vi "Write Single Holding Register.vi"(8 "error in (no error)":errorcluster, 9 "register to write":u16, 10 "address":u16, 11 "Modbus instance in":refnum<class "Modbus API.lvclass">) -> (0 "error out":errorcluster, 3 "Modbus instance out":refnum<class "Modbus API.lvclass">)   [LabVIEW 2020, in "SubVIs.lvlib" / "Modbus API.lvclass"]
doc: "Writes <B>register to write</B> to <B>address</B> of the device."
uses:
  <vilib>/Modbus/subvis/Modbus API/Modbus API.lvclass
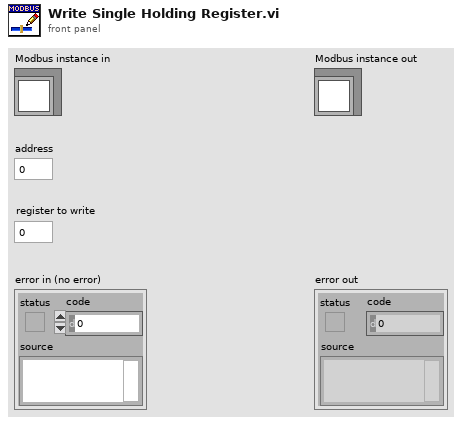
[diagram p1: front panel]
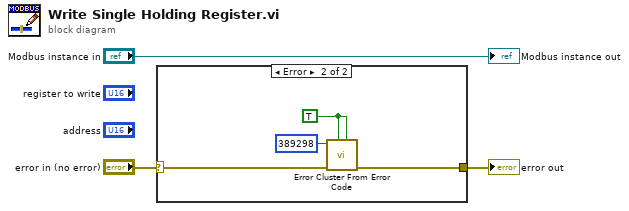
[diagram p0: block diagram]
diagram:
  n1 = case shown="Error" "error in (no error)" {
    selector: "error in (no error)" -> [w4 w7]
    tunnel: [w4 w8] -> w1
    frame No Error {
    }
    frame Error {
      w5 = TRUE ("show call chain? (False)")
      n2 = call <vilib>:"Error Cluster From Error Code.vi"("is warning? (False)"=w5, "show call chain? (False)"=w5, "error in (no error)"=w7, "error code (0)"=389298) -> ("error out"=w8:errorcluster)  [unwired: 5 in]
    }
  }
  "error out" <- w1
  "Modbus instance out" <- "Modbus instance in"
